vi "Find Static Test Methods in Test Case.vi"(8 "error in (no error)":errorcluster, 10 "Test Case Class Path":path, 11 "Indexing Test Finder In":refnum<class "Indexing Test Finder.lvclass">) -> (0 "error out":errorcluster, 2 "Test Methods Out":map{string, path}(c390), 3 "Indexing Test Finder Out":refnum<class "Indexing Test Finder.lvclass">)   [LabVIEW 2020, in "Indexing Test Finder.lvclass"]
uses:
  Indexing Test Finder.lvclass
  Indexing Test Finder.lvclass/Indexing Test Finder.ctl
  Test Finder/Test Finder.lvclass
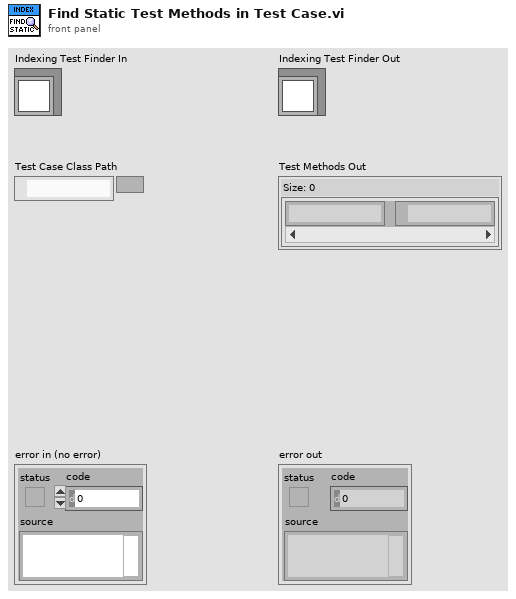
[diagram p1: front panel]
types:
  T1 = typedef "Indexing Test Finder.lvclass/Index Item.ctl" = cluster{"Dynamic Methods":map{string, path}, "Static Methods":map{string, path}, "Signature":string}
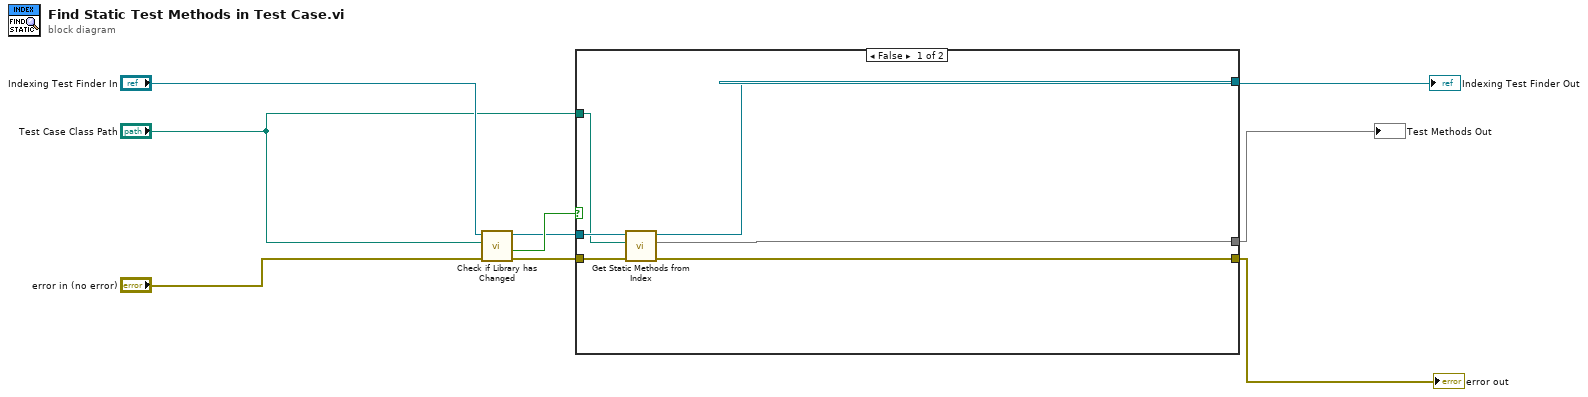
[diagram p0: block diagram]
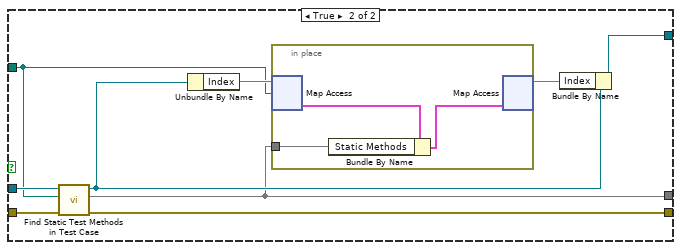
[diagram p2: hidden frame]
diagram:
  n1 = call "Check if Library has Changed.vi"("error in (no error)"="error in (no error)", "Test Case Path"="Test Case Class Path", "Indexing Test Finder in"="Indexing Test Finder In") -> ("error out"=w1:errorcluster, "Index out of date?"=w3:bool, "Indexing Test Finder out"=w2:refnum<class "Indexing Test Finder.lvclass">)  [unwired: 6 in]
  n2 = case shown="False" w3 {
    tunnel: w2 -> [w15 w24]
    tunnel: w1 -> [w14 w23]
    tunnel: "Test Case Class Path" -> [w13 w16]
    tunnel: [w10 w20] -> w7
    tunnel: [w12 w17] -> w8
    tunnel: [w11 w22] -> w9
    frame False {
      n3 = call "Get Static Methods from Index.vi"("error in (no error)"=w14, "Test Case Class Path"=w13, "Indexing Test Finder in"=w15) -> ("error out"=w11:errorcluster, "Test Methods"=w12:map{string, path}, "Indexing Test Finder out"=w10:refnum<class "Indexing Test Finder.lvclass">)  [unwired: 6 in]
    }
    frame True {
      n4 = call-parent "Find Static Test Methods in Test Case.vi"("error in (no error)"=w23, "Test Case Class Path"=w16, "Test Finder In"=w24) -> ("error out"=w22:errorcluster, "Test Methods Out"=w17:map{string, path}, "Test Finder Out"=w18:refnum<class "Indexing Test Finder.lvclass">)  [unwired: 6 in]
      n5 = Unbundle By Name(w18) -> ("Index"=w21:map{path, T1})
      n6 = in-place "In Place Element Structure" {
        in-place-border: w17 -> [w25]
        n7 = in-place-map #1(w21, w16) -> (w27:T1)  [unwired: 1 in, 1 out]
        n8 = Bundle By Name(cluster=w27, "Static Methods"=w25) -> (w26:T1)
        n9 = in-place-map #1(w26) -> (w19:map{path, T1})  [unwired: 1 in, 2 out]
      }
      n10 = Bundle By Name(cluster=w18, "Index"=w19) -> (w20:refnum<class "Indexing Test Finder.lvclass">)
    }
  }
  "error out" <- w9
  "Test Methods Out" <- w8
  "Indexing Test Finder Out" <- w7
